vi "Meas Get Record Section - Make Groups.vi"(5 "max group size (2)":i32=2, 7 "waveforms group selector ref":refnum<vi>, 8 "error in (no error)":errorcluster, 10 "all labels":string[](array[string]), 11 "all waveforms in [V]":sgl[][](array[numeric])) -> (0 "error out":errorcluster, 2 "selected labels":string[](array[string]), 3 "selected waveforms out [V]":sgl[][](array[numeric]))   [LabVIEW 2020]
doc: "Makes and selects waveforms groups based on transducer mapping. E.g. combines u1+i1, u2+i2, u1+u2+u3, etc. This is intended as subvi of Meas Get Record Section.vi."
uses:
  a171010d-f420-478d-8c15-a35804a7db7e.vi
  a4db784f-2cf2-4c9e-9619-b3011bc32df0.vi
  ba0b6a6c-8790-4ffc-a797-b51ada32875d.vi
  11fe3a4c-4f3e-4b8e-9818-3b3cacd1e437.vi
  cde7318f-3917-455b-8ebc-3fa5aa8aefe8.vi
  3982fa26-95e5-4eb8-b606-bf7940dc71af.vi
  <vilib>/regexp/Match Regular Expression.xnode
  <vilib>/Comparison/Equal/Equal Functor/Equal Functor.lvclass
panel:
  out "menu":string[](array[string])
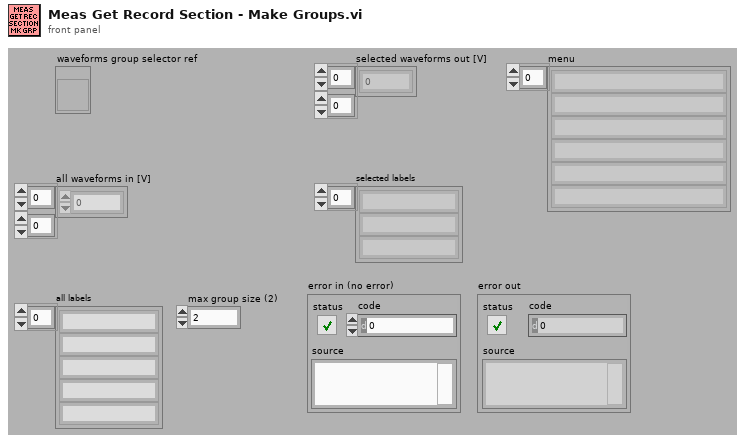
[diagram p1: front panel]
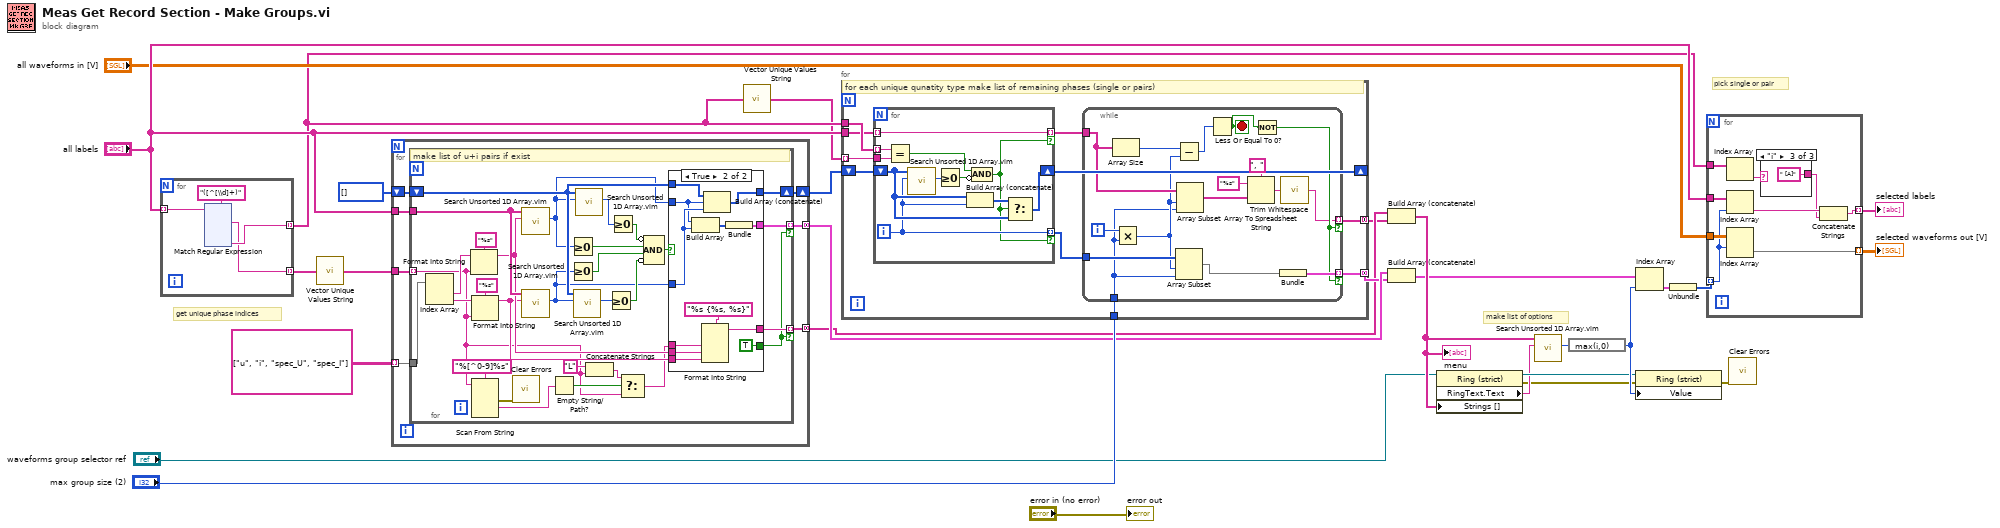
[diagram p0: block diagram]
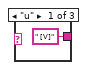
[diagram p3: hidden frame]
diagram:
  # "make list of options"
  # "pick single or pair"
  # "get unique phase indices"
  n1 = for {
    tunnel: "all labels" -> [w32] mode=indexing
    tunnel: [w29] -> w3 mode=indexing
    tunnel: [w31] -> w5 mode=indexing
    n2 = xnode "Match Regular Expression"("input string"=w32, "regular expression"="([^[\\d]+)" ("format string")) -> ("after match"=w29:string, "submatch 1"=w31:string)  [unwired: 4 in, 4 out]
  }
  n3 = call "Vector Unique Values String.vi"("array in"=w3) -> ("uniques out"=w2:string[])
  n4 = for {
    tunnel: "all labels" -> [w155]
    tunnel: [w154] -> w13 mode=concatenating
    tunnel: [w153] -> w11 mode=concatenating
    tunnel: w2 -> [w150]
    shift-right: [w152] -> w9
    shift-left: i32[] [] -> [w151]
    tunnel: string[][] [["u", "i"], ["spec_U", "spec_I"]] -> [w149] mode=indexing
    n5 = for {
      tunnel: w150 -> [w157] mode=indexing
      tunnel: w155 -> [w183]
      shift-right: [w171] -> w152
      shift-left: w151 -> [w172]
      tunnel: [w173] -> w153 mode=indexing if=w167
      tunnel: [w168] -> w154 mode=indexing if=w167
      tunnel: w149 -> [w166]
      # "make list of u+i pairs if exist"
      n6 = Index Array(array=w166) -> (element #1=w164:string, element #2=w165:string)  [unwired: 2 in]
      n7 = Format Into String(format string="%s", initial string=w164, w157) -> (resulting string=w175:string)  [unwired: 1 in, 1 out]
      n8 = Format Into String(format string="%s", initial string=w165, w157) -> (resulting string=w174:string)  [unwired: 1 in, 1 out]
      n9 = Scan From String(format string="%[^0-9]%s", input string=w157) -> (error out=w162:errorcluster, output 1=w160:string)  [unwired: 5 in, 2 out]
      n10 = call <vilib>:"Clear Errors.vi"("error in (no error)"=w162) -> ()  [unwired: 5 in, 2 out]
      n11 = call "Search Unsorted 1D Array.vim"("element"=w175, "unsorted 1D array"=w183) -> ("index of element"=w169:i32)  [unwired: 9 in]
      n12 = call "Search Unsorted 1D Array.vim"("element"=w174, "unsorted 1D array"=w183) -> ("index of element"=w170:i32)  [unwired: 9 in]
      n13 = Empty String/Path?(string/path=w160) -> (empty?=w161:bool)
      n14 = Greater Or Equal To 0?(x=w169) -> (x >= 0?=w182:bool)
      n15 = Greater Or Equal To 0?(x=w170) -> (x >= 0?=w181:bool)
      n16 = call "Search Unsorted 1D Array.vim"("element"=w170, "unsorted 1D array"=w172) -> ("index of element"=w178:i32)  [unwired: 9 in]
      n17 = call "Search Unsorted 1D Array.vim"("element"=w169, "unsorted 1D array"=w172) -> ("index of element"=w180:i32)  [unwired: 9 in]
      n18 = Concatenate Strings("L" ("string"), w157) -> (w159:string)
      n19 = Greater Or Equal To 0?(x=w178) -> (x >= 0?=w177:bool)
      n20 = Greater Or Equal To 0?(x=w180) -> (x >= 0?=w179:bool)
      n21 = Select(t=w159, s=w161, f=w157) -> (s? t:f=w156:string)
      n22 = Compound Arithmetic op=AND(invert w179, w182, w181, invert w177) -> (w176:bool)
      n23 = case shown="True" w176 {
        tunnel: w156 -> [_ w197]
        tunnel: w175 -> [_ w196]
        tunnel: w174 -> [_ w195]
        tunnel: [_ w194] -> w173
        tunnel: w172 -> [w186 w193]
        tunnel: [w186 w192] -> w171
        tunnel: w170 -> [_ w190]
        tunnel: w169 -> [_ w189]
        tunnel: [_ TRUE] -> w167
        tunnel: [_ w187] -> w168
        frame False {
        }
        frame True {
          n24 = Build Array(w189, w190) -> (w188:i32[])
          n25 = Format Into String(format string="%s {%s, %s}", w197, w196, w195) -> (resulting string=w194:string)  [unwired: 2 in, 1 out]
          n26 = Build Array (concatenate)(w193, w189, w190) -> (w192:i32[])
          n27 = Bundle(w188) -> (w187:cluster{i32[]})  [unwired: 1 in]
        }
      }
    }
  }
  n28 = call "Vector Unique Values String.vi"("array in"=w5) -> ("uniques out"=w4:string[])
  n29 = for {
    tunnel: "all labels" -> [w205]
    tunnel: w4 -> [w208] mode=indexing
    tunnel: w5 -> [w207]
    shift-right: [w204] -> _
    shift-left: w9 -> [w206]
    tunnel: [w201] -> w10 mode=concatenating
    tunnel: [w200] -> w12 mode=concatenating
    tunnel: "max group size (2)" -> [w199]
    # "for each unique qunatity type make list of remaining phases (single or pairs)"
    n30 = for {
      tunnel: w208 -> [w235]
      tunnel: w207 -> [w234] mode=indexing
      tunnel: w205 -> [w230] mode=indexing
      tunnel: [w230] -> w203 mode=indexing if=w225
      shift-right: [w229] -> w204
      shift-left: w206 -> [w228]
      tunnel: [w226] -> w202 mode=indexing if=w225
      i -> [w226]
      n31 = Equal?(x=w234, y=w235) -> (x = y?=w233:bool)
      n32 = call "Search Unsorted 1D Array.vim"("element"=w226, "unsorted 1D array"=w228) -> ("index of element"=w232:i32)  [unwired: 9 in]
      n33 = Greater Or Equal To 0?(x=w232) -> (x >= 0?=w231:bool)
      n34 = Build Array (concatenate)(w228, w226) -> (w227:i32[])
      n35 = Compound Arithmetic op=AND(w233, invert w231) -> (w225:bool)
      n36 = Select(t=w227, s=w225, f=w228) -> (s? t:f=w229:i32[])
    }
    n37 = while {
      tunnel: w203 -> [w218]
      tunnel: [w213] -> w201 mode=indexing if=w221
      tunnel: w202 -> [w212]
      tunnel: [w222] -> w200 mode=indexing if=w221
      tunnel: w199 -> [w210]
      i -> [w220]
      stop <- w223 stop-if-true
      n38 = Array Size(array=w218) -> (size(s)=w224:i32)
      n39 = Multiply(x=w220, y=w210) -> (x*y=w211:i32)
      n40 = Subtract(x=w224, y=w211) -> (x-y=w219:i32)
      n41 = Array Subset(array=w212, index=w211, length=w210) -> (w209:i32[])
      n42 = Array Subset(array=w218, index=w211, length=w210) -> (w217:string[])
      n43 = Less Or Equal To 0?(x=w219) -> (x <= 0?=w223:bool)
      n44 = Array To Spreadsheet String(delimiter (Tab)=", ", array=w217, 3:"%s" ("format string")) -> (spreadsheet string=w214:string)
      n45 = Not(x=w223) -> (.not. x?=w221:bool)
      n46 = Bundle(w209) -> (w222:cluster{i32[]})  [unwired: 1 in]
      n47 = call <vilib>:"Trim Whitespace.vi"("string"=w214) -> ("trimmed string"=w213:string)  [unwired: 1 in]
    }
  }
  n48 = Build Array (concatenate)(w11, w10) -> (w23:string[])
  "menu" <- w23
  n49 = Build Array (concatenate)(w13, w12) -> (w19:cluster{i32[]}[])
  n50 = property class="Ring (strict)"(reference="waveforms group selector ref", "Strings []"=w23) -> (reference out=w17:refnum<vi>, error out=w6:errorcluster, "RingText.Text"=w15:string)  [unwired: 1 in]
  n51 = call "Search Unsorted 1D Array.vim"("element"=w15, "unsorted 1D array"=w23) -> ("index of element"=w16:i32)  [unwired: 9 in]
  n52 = expression code="max(i,0)"(w16) -> (w24:i32)
  n53 = Index Array(array=w19, index=w24) -> (element=w20:cluster{i32[]})
  n54 = property class="Ring (strict)"(reference=w17, error in=w6, "Value"=w24) -> (error out=w18:errorcluster)  [unwired: 1 out]
  n55 = Unbundle(w20) -> (w21:i32[])
  n56 = for {
    tunnel: w21 -> [w241] mode=indexing
    tunnel: "all waveforms in [V]" -> [w244]
    tunnel: [w243] -> w25 mode=indexing
    tunnel: "all labels" -> [w242]
    tunnel: [w237] -> w27 mode=indexing
    tunnel: w5 -> [w240]
    n57 = Index Array(array=w240) -> (element=w239:string)  [unwired: 1 in]
    n58 = Index Array(array=w242, index=w241) -> (element=w238:string)
    n59 = Index Array(array=w244, index (row)=w241) -> (element=w243:sgl[])  [unwired: 1 in]
    n60 = case shown="\"i\"" w239 {
      tunnel: [" [V]" _ " [A]"] -> w236
      frame "u" {
      }
      frame Default {
      }
      frame "i" {
      }
    }
    n61 = Concatenate Strings(w238, w236) -> (w237:string)
  }
  "selected labels" <- w27
  "selected waveforms out [V]" <- w25
  n62 = call <vilib>:"Clear Errors.vi"("error in (no error)"=w18) -> ()  [unwired: 5 in, 2 out]
  "error out" <- "error in (no error)"
